vi "Clear Serial Port.vi"(8 "error in (no error)":errorcluster, 11 "Listener In.lvclass":refnum<class "Listener.lvclass">) -> (0 "error out":errorcluster, 3 "Listener out":refnum<class "Listener.lvclass">)   [LabVIEW 2023, in "Listener.lvclass"]
doc: "Calls Visa Clear on the specified COM port"
uses:
  Listener.lvclass
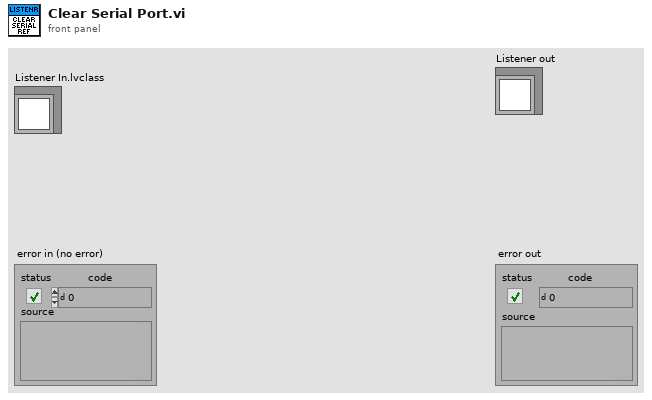
[diagram p1: front panel]
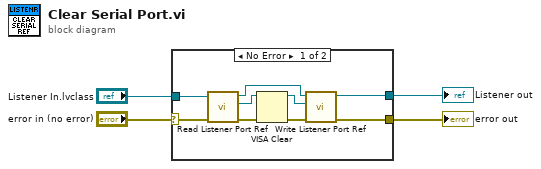
[diagram p0: block diagram]
diagram:
  n1 = case shown="No Error" "error in (no error)" {
    selector: "error in (no error)" -> [w12 w15]
    tunnel: [w11 w15] -> w3
    tunnel: "Listener In.lvclass" -> [w13 w14]
    tunnel: [w10 w14] -> w1
    frame No Error {
      n2 = call "Read Listener Port Ref.vi"("error in (no error)"=w12, "Listener in"=w13) -> ("error out"=w9:errorcluster, "Listener Port Ref"=w8:refnum<visa-resource-name>, "Listener out"=w5:refnum<class "Listener.lvclass">)  [unwired: 7 in]
      n3 = VISA Clear(VISA resource name=w8, error in (no error)=w9) -> (VISA resource name out=w6:refnum<visa-resource-name>, error out=w7:errorcluster)
      n4 = call "Write Listener Port Ref.vi"("error in (no error)"=w7, "Listener Port Ref"=w6, "Listener in"=w5) -> ("error out"=w11:errorcluster, "Listener out"=w10:refnum<class "Listener.lvclass">)  [unwired: 7 in]
    }
    frame Error {
    }
  }
  "error out" <- w3
  "Listener out" <- w1
